vi "Set Stamp Tool Vacuum.vi"(8 "error in":errorcluster, 9 "On/Off":bool, 11 "Gantry in":refnum<class "Gantry Class.lvclass">) -> (0 "error out":errorcluster, 3 "Gantry out":refnum<class "Gantry Class.lvclass">)   [LabVIEW 2011, in "Gantry Class.lvclass"]
uses:
  Gantry Class.lvclass
  WorkTable Class/WorkTable Class.lvclass
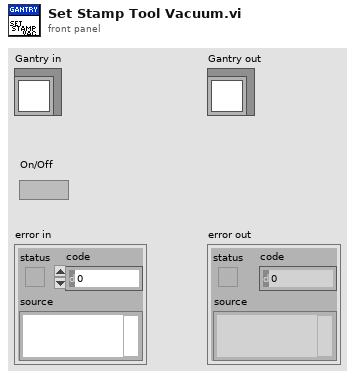
[diagram p1: front panel]
types:
  T1 = typedef "Worktable_Stamps.ctl" = cluster{"Stamp Slots":cluster{"Stamp State":enum16{"Empty", "Populated", "Used"}, "Stamp Type":enum16{"Stamp 1", "Stamp 2", "Stamp 3", "Stamp 4"}, "Location/Orientation":T2}[], "Vacuum Channel":u8}
  T2 = typedef "Position_Orientation.ctl" = cluster{"Center":refnum<class "Vec3d Class.lvclass">, "Orientation":refnum<class "Orient3d Class.lvclass">}
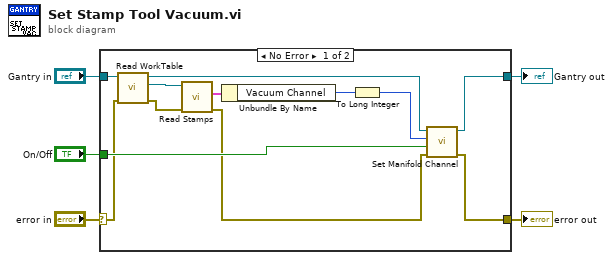
[diagram p0: block diagram]
diagram:
  n1 = case shown="No Error" "error in" {
    selector: "error in" -> [w9 w19]
    tunnel: [w13 w19] -> w3
    tunnel: [w14 w18] -> w4
    tunnel: "Gantry in" -> [w17 w18]
    tunnel: "On/Off" -> [w16 _]
    frame No Error {
      n2 = call-dynamic "Read WorkTable.vi"("error in"=w9, "Gantry Class in"=w17) -> ("error out"=w10:errorcluster, "WorkTable Class.lvclass"=w12:refnum<class "WorkTable Class.lvclass">, "Gantry Class out"=w15:refnum<class "Gantry Class.lvclass">)  [unwired: 7 in]
      n3 = call-dynamic "Read Stamps.vi"("error in (no error)"=w10, "WorkTable Class in"=w12) -> ("error out"=w8:errorcluster, "Stamps"=w11:T1)  [unwired: 7 in, 1 out]
      n4 = Unbundle By Name(w11) -> ("Vacuum Channel"=w7:u8)
      n5 = To Long Integer(number=w7) -> (32bit integer=w6:i32)
      n6 = call-dynamic "Set Manifold Channel.vi"("error in"=w8, "On/Off"=w16, "Manifold Channel"=w6, "Gantry in"=w15) -> ("error out"=w13:errorcluster, "Gantry out"=w14:refnum<class "Gantry Class.lvclass">)  [unwired: 6 in]
    }
    frame Error {
    }
  }
  "error out" <- w3
  "Gantry out" <- w4
